vi "CalculoTesteSenoide_Validacao.vi"(9 "Rotações por minuto":dbl, 10 "Min":dbl, 11 "Max":dbl) -> (3 "XY Graph":cluster{"X":dbl, "Y":dbl}[](graph))   [LabVIEW 2019]
uses:
  <vilib>/Analysis/NI_AAL_SigProc.lvlib
panel:
  out "Array":dbl[](array[numeric])
  # "Max: 60 pontos por segundo"
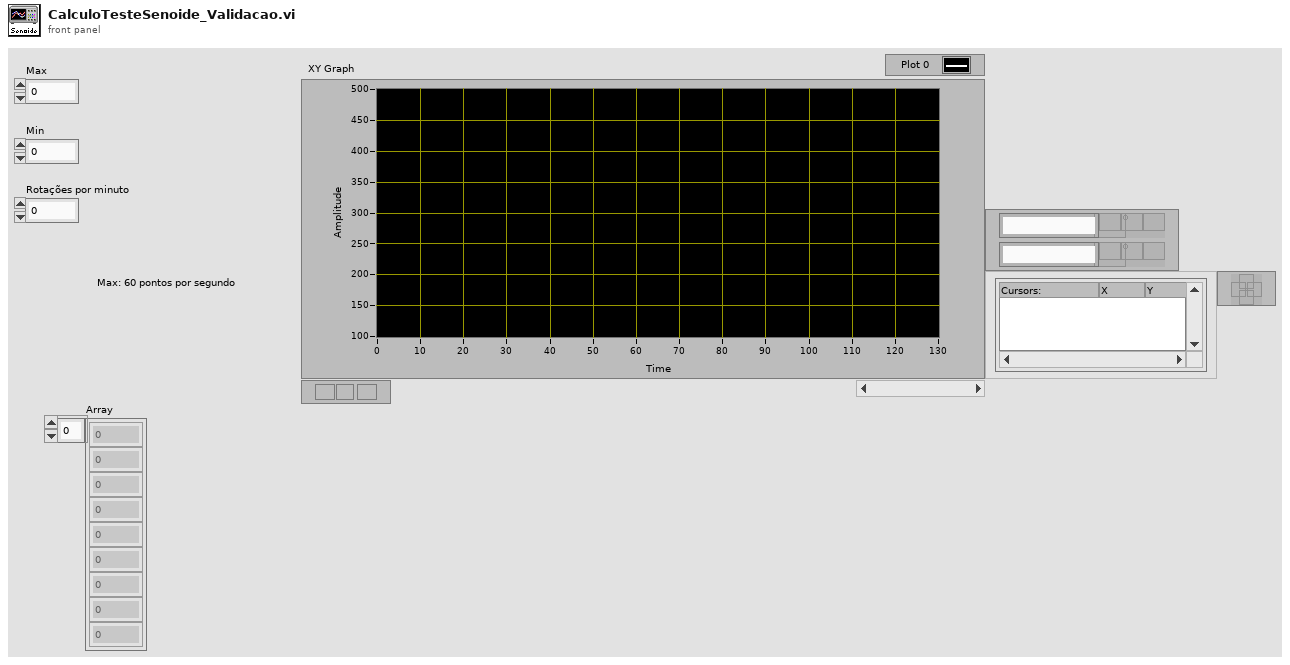
[diagram p1: front panel]
types:
  T1 = cluster{"RotaçãoPorSeg":dbl, "Fase":dbl, "AmplitudeOnda":dbl, "Offset":dbl}
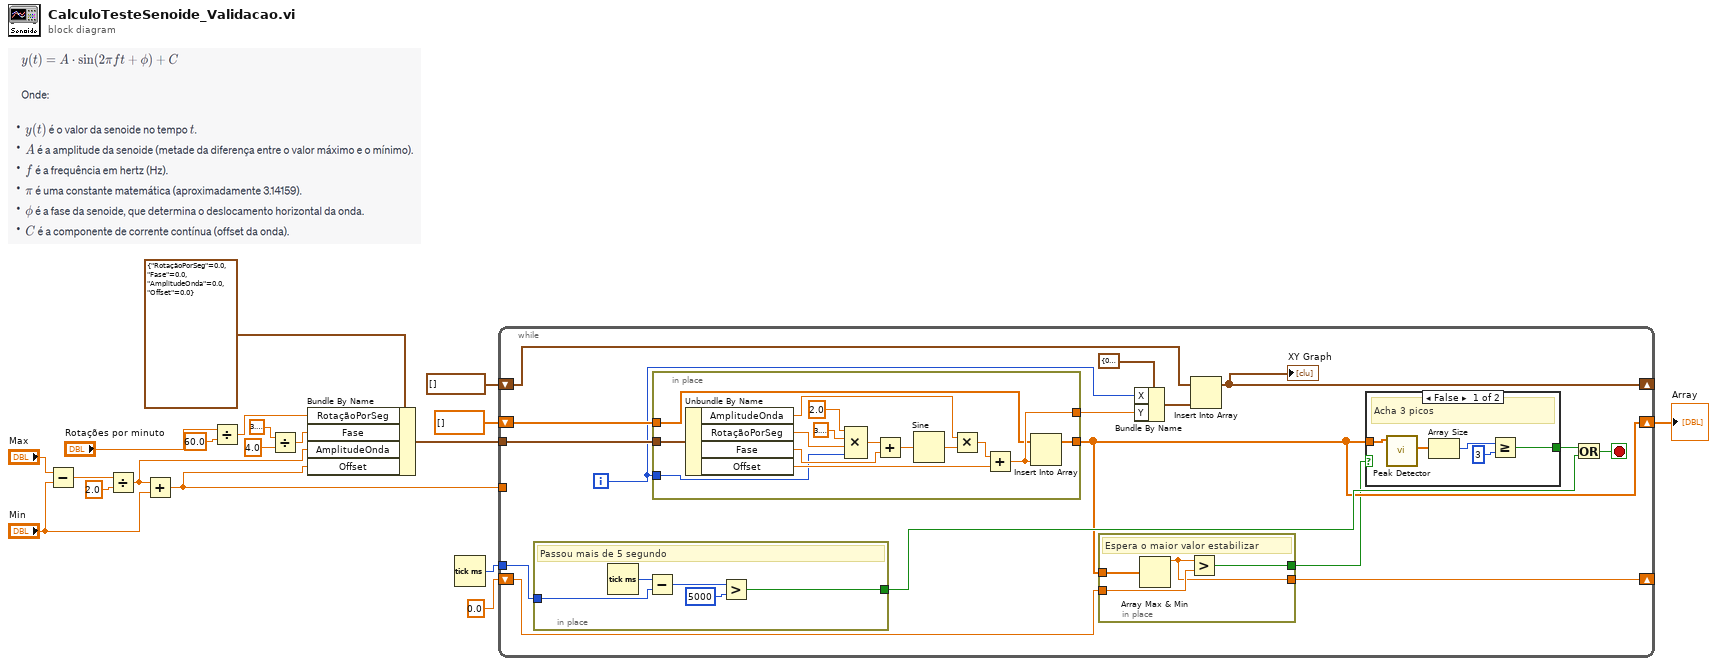
[diagram p0: block diagram]
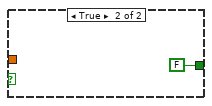
[diagram p2: hidden frame]
diagram:
  n1 = Subtract(x="Max", y="Min") -> (x-y=w10:dbl)
  n2 = Divide(x=w10, y=2.0) -> (x/y=w5:dbl)
  n3 = Add(x=w5, y="Min") -> (x+y=w1:dbl)
  n4 = Divide(x="Rotações por minuto", y=60.0) -> (x/y=w7:dbl)
  n5 = Divide(x=3.141592653589793, y=4.0) -> (x/y=w6:dbl)
  n6 = Bundle By Name(cluster=T1 {"RotaçãoPorSeg"=0.0, "Fase"=0.0, "AmplitudeOnda"=0.0, "Offset"=0.0}, "RotaçãoPorSeg"=w7, "Fase"=w6, "AmplitudeOnda"=w5, "Offset"=w1) -> (w4:T1)
  n7 = Tick Count (ms)() -> (millisecond timer value=w11:u32)
  n8 = while {
    shift-right: [w26] -> w2
    shift-left: dbl[] [] -> [w27]
    shift-right: [w34] -> _
    shift-left: cluster{"X":dbl, "Y":dbl}[] [] ("GraphSenoide") -> [w35]
    tunnel: w11 -> [w30]
    shift-right: [w23] -> _
    shift-left: 0.0 -> [w25]
    tunnel: w4 -> [w21]
    tunnel: w1 -> [_]
    i -> [w20]
    stop <- w28 stop-if-true
    n9 = in-place {
      in-place-border: w30 -> [w65]
      in-place-border: [w61] -> w29
      # "Passou mais de 5 segundo"
      n10 = Tick Count (ms)() -> (millisecond timer value=w64:u32)
      n11 = Subtract(x=w64, y=w65) -> (x-y=w63:u32)
      n12 = Greater?(x=w63, y=u32 5000) -> (0:w61:bool)
    }
    n13 = in-place {
      in-place-border: [w44] -> w31
      in-place-border: w27 -> [w43]
      in-place-border: [w42] -> w26
      in-place-border: w21 -> [w41]
      in-place-border: w20 -> [w36]
      n14 = Unbundle By Name(w41) -> ("AmplitudeOnda"=w38:dbl, "RotaçãoPorSeg"=w40:dbl, "Fase"=w39:dbl, "Offset"=w37:dbl)
      n15 = Compound Arithmetic op=MULTIPLY(2.0, 3.141592653589793, w40, w36) -> (w47:dbl)
      n16 = Add(x=w47, y=w39) -> (x+y=w46:dbl)
      n17 = Sine(x=w46) -> (sin(x)=w48:dbl)
      n18 = Multiply(x=w38, y=w48) -> (x*y=w45:dbl)
      n19 = Add(x=w45, y=w37) -> (x+y=w44:dbl)
      n20 = Insert Into Array(array=w43, new element=w44) -> (w42:dbl[])  [unwired: 1 in]
    }
    n21 = in-place {
      in-place-border: w26 -> [w54]
      in-place-border: w25 -> [w53]
      in-place-border: [w52] -> w24
      in-place-border: [w51] -> w23
      # "Espera o maior valor estabilizar"
      n22 = Array Max & Min(array=w54) -> (max value=w51:dbl)  [unwired: 3 out]
      n23 = Greater?(x=w51, y=w53) -> (0:w52:bool)
    }
    n24 = Bundle By Name(cluster=cluster{"X":dbl, "Y":dbl} {"X"=0.0, "Y"=0.0} ("new element/subarray"), "X"=w20, "Y"=w31) -> (w32:cluster{"X":dbl, "Y":dbl})
    n25 = Insert Into Array(array=w35, new element=w32) -> (w34:cluster{"X":dbl, "Y":dbl}[])  [unwired: 1 in]
    "XY Graph" <- w34
    n26 = case shown="False" w24 {
      tunnel: w26 -> [w59 _]
      tunnel: [w55 FALSE] -> w22
      frame False {
        # "Acha 3 picos"
        n27 = call <vilib>:"Peak Detector.vi"("X"=w59) -> ("Amplitudes"=w56:dbl[])  [unwired: 6 in, 4 out]
        n28 = Array Size(array=w56) -> (size(s)=w58:i32)
        n29 = Greater Or Equal?(x=w58, y=3) -> (x >= y?=w55:bool)
      }
      frame True {
      }
    }
    n30 = Or(x=w22, y=w29) -> (x .or. y?=w28:bool)
  }
  "Array" <- w2
